vi "_Remote Park Lens.vi"(4 "error in":errorcluster, 7 "All Ch (F)":bool) -> (0 "error out":errorcluster)   [LabVIEW 2015]
uses:
  Type/_RT Active Ch.ctl
  Configuration/_Global Configuration.vi
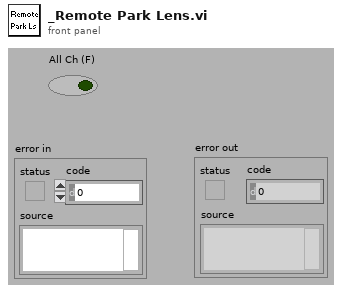
[diagram p1: front panel]
types:
  T1 = typedef "_RT Active Ch.ctl" = cluster{"Start":i32, "Step":i32, "ChID":i32}
  T2 = typedef "_RT Instrument 2.ctl" = cluster{"Table":T3[], "Instrument":string[]}
  T3 = typedef "_RT Configuration 2.ctl" = cluster{"Name":string, "Ch#":u8, "Min":dbl, "Max":dbl, "Def+":dbl, "Def-":dbl, "Offset":dbl, "Slope":dbl, "Type":u8, "Description":string, "SettleT":dbl}
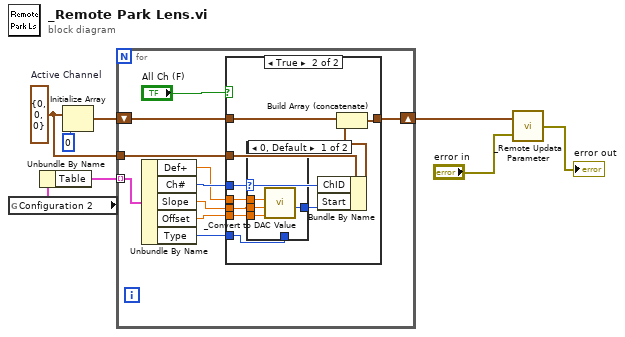
[diagram p0: block diagram]
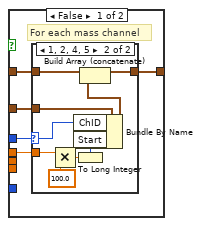
[diagram p2: hidden frame]
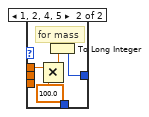
[diagram p4: hidden frame]
diagram:
  w4 = T1 {"Start"=0, "Step"=0, "ChID"=0}  # Active Channel
  n1 = global read "_Global Configuration.vi" "Configuration 2"() -> (w7:T2)
  n2 = Unbundle By Name(w7) -> ("Table"=w8:T3[])
  n3 = Initialize Array(w4, 0 ("dimension size")) -> (w5:T1[])
  n4 = for {
    tunnel: w8 -> [w17] mode=indexing
    shift-right: [w14] -> w3
    shift-left: w5 -> [w15]
    tunnel: w4 -> [w13]
    n5 = Unbundle By Name(w17) -> ("Def+"=w16:dbl, "Ch#"=w18:u8, "Slope"=w11:dbl, "Offset"=w10:dbl, "Type"=w9:u8)
    n6 = case shown="True" "All Ch (F)" {
      tunnel: w18 -> [w23 w39]
      tunnel: w16 -> [w22 w37]
      tunnel: w15 -> [w21 w43]
      tunnel: [w20 w42] -> w14
      tunnel: w13 -> [w19 w41]
      tunnel: w11 -> [_ w36]
      tunnel: w10 -> [_ w35]
      tunnel: w9 -> [_ w34]
      frame False {
        # "For each mass channel"
        n7 = case shown="1, 2, 4, 5" w23 {
          selector: w23 -> [_ w29]
          tunnel: w22 -> [_ w33]
          tunnel: w21 -> [w24 w27]
          tunnel: [w24 w26] -> w20
          tunnel: w19 -> [_ w28]
          frame 0, Default {
          }
          frame 1, 2, 4, 5 {
            n8 = Multiply(x=w33, y=100.0) -> (x*y=w31:dbl)
            n9 = To Long Integer(number=w31) -> (32bit integer=w30:i32)
            n10 = Bundle By Name(cluster=w28, "ChID"=w29, "Start"=w30) -> (w25:T1)
            n11 = Build Array (concatenate)(w27, w25) -> (w26:T1[])
          }
        }
      }
      frame True {
        n12 = case shown="0, Default" w39 {
          selector: w39 -> [w44 _]
          tunnel: w37 -> [w48 w52]
          tunnel: w36 -> [w47 _]
          tunnel: w35 -> [w46 _]
          tunnel: [w45 w49] -> w38
          tunnel: w34 -> [_ _]
          frame 0, Default {
            n13 = call "_Convert to DAC Value.vi"("Offset"=w46, "Slop"=w47, "Number"=w48, "Channel"=w44) -> ("DAC Value"=w45:i32)  [unwired: 3 in, 4 out]
          }
          frame 1, 2, 4, 5 {
            # "for mass"
            n14 = Multiply(x=w52, y=100.0) -> (x*y=w50:dbl)
            n15 = To Long Integer(number=w50) -> (32bit integer=w49:i32)
          }
        }
        n16 = Bundle By Name(cluster=w41, "ChID"=w39, "Start"=w38) -> (w40:T1)
        n17 = Build Array (concatenate)(w43, w40) -> (w42:T1[])
      }
    }
  }
  n18 = call "_Remote Updata Parameter.vi"("error in"="error in", "Parameters"=w3) -> ("error out"=→"error out":errorcluster)
